vi "Poly Fit Clipped Data.vi"(0 "Intensity Data":dbl[](array[numeric])=[5.666666666666668, 2.666666666666668, -0.33333333333333215, 0.6666666666666679, -2.333333333333332, -5.333333333333332, -2.333333333333332, -4.333333333333332, -4.333333333333332, -0.33333333333333215, 0.6666666666666679, 2.666666666666668, 3.666666666666668, 12.666666666666668, 11.666666666666668, 16.666666666666668, 19.666666666666668, 25.666666666666668, 35.66666666666667, 46.66666666666667, 76.66666666666667, 119.66666666666667, 169.66666666666666, 227.66666666666666, 227.66666666666666, 227.66666666666666, 227.66666666666666, 227.66666666666666, 227.66666666666666, 130.66666666666666, 67.66666666666667, 26.666666666666668, 17.666666666666668, 11.666666666666668, 5.666666666666668, 4.666666666666668, 7.666666666666668, 4.666666666666668, 2.666666666666668, -2.333333333333332, -2.333333333333332, -3.333333333333332, -4.333333333333332, -3.333333333333332, -4.333333333333332, -2.333333333333332, -2.333333333333332, 0.6666666666666679, 0.6666666666666679, -0.33333333333333215]) -> ()   [LabVIEW 2012]
uses:
  <userlib>/_OpenG.lib/array/array.llb/Slice 1D Array (DBL)__ogtk.vi
  <vilib>/Analysis/polynomials.llb/Polynomial Plot (Samples).vi
  <vilib>/Analysis/NI_AALPro.lvlib
panel:
  out "amplitude":dbl
  out "error out":errorcluster
  in  "slice":string
  out "Observed Data and Fitted Curve  2":cluster{cluster{"Numeric":dbl, "p(x)":dbl}[]}[](graph) caption="Observed Data and Fitted Curve"
  in  "polynomial order":i32=2
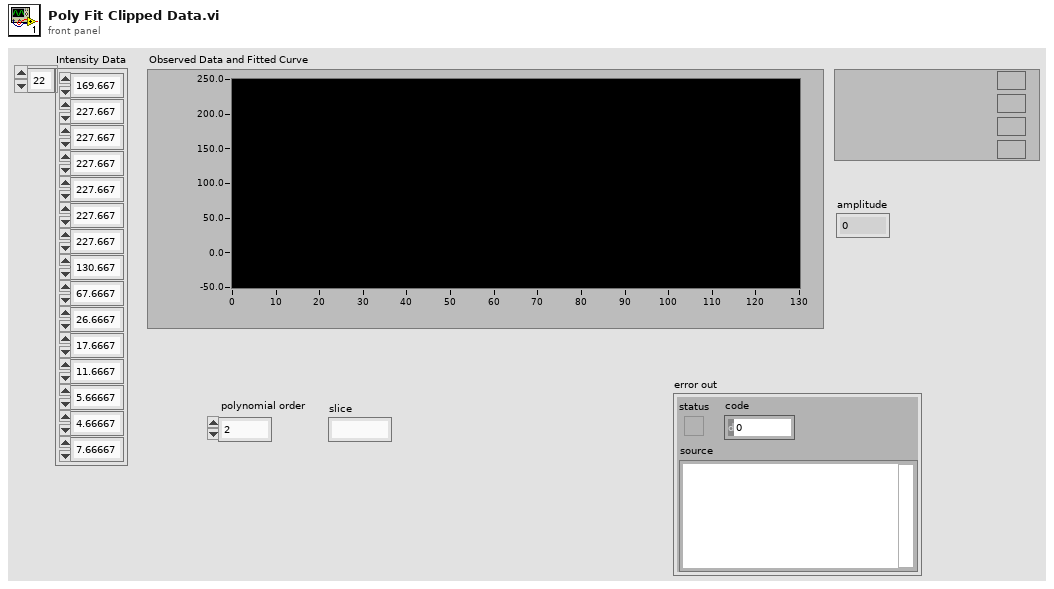
[diagram p1: front panel]
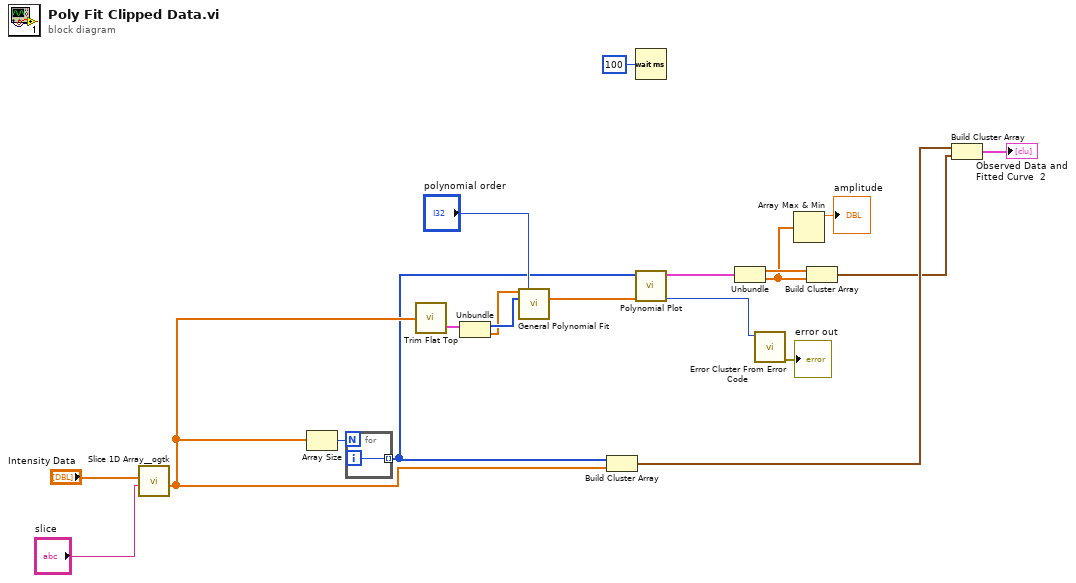
[diagram p0: block diagram]
diagram:
  n1 = call-poly <userlib>:"Slice 1D Array__ogtk.vi"("slice"="slice", "array"="Intensity Data") -> ("subarray (array[i:j])"=w11:dbl[])  [unwired: 5 in]
  n2 = Array Size(array=w11) -> (size(s)=w13:i32)
  n3 = for {
    N: w13 -> [_]
    tunnel: [w21] -> w8 mode=indexing
    i -> [w21]
  }
  n4 = call "Trim Flat Top.vi"("Data In"=w11) -> ("Trimmed Data (x,y)"=w18:cluster{i32[], dbl[]})  [unwired: 1 out]
  n5 = Unbundle(w18) -> (w17:i32[], w16:dbl[])
  n6 = call <vilib>:"General Polynomial Fit.vi"("Y"=w16, "polynomial order"="polynomial order", "X"=w17) -> ("Polynomial Coefficients"=w9:dbl[])  [unwired: 9 in, 3 out]
  n7 = Build Cluster Array(w8, w11) -> (w15:cluster{i32, "Numeric":dbl}[])
  n8 = Wait (ms)(milliseconds to wait=u32 100) -> ()  [unwired: 1 out]
  n9 = call-poly <vilib>:"Polynomial Plot.vi"("P(x)"=w9, "X"=w8) -> ("error"=w4:i32, "polynomial plot"=w7:cluster{dbl[], "P(A)":dbl[]})  [unwired: 8 in]
  n10 = Unbundle(w7) -> (w6:dbl[], "P(A)"=w2:dbl[])
  n11 = call <vilib>:"Error Cluster From Error Code.vi"("error code (0)"=w4) -> ("error out"=→"error out":errorcluster)  [unwired: 8 in]
  n12 = Array Max & Min(array=w2) -> (max value=→"amplitude":dbl)  [unwired: 3 out]
  n13 = Build Cluster Array(w6, w2) -> (w5:cluster{"Numeric":dbl, "p(x)":dbl}[])
  n14 = Build Cluster Array(w15, w5) -> (→"Observed Data and Fitted Curve  2":cluster{cluster{"Numeric":dbl, "p(x)":dbl}[]}[])
